vi "FPGA-7841R-Control V3.vi"(0 "Waveform Data":T4, 1 "Current Frame":u8, 2 "Action":T5=enum."Exit", 3 "Laser On Time (Ticks)":u8=13, 5 "Laser Controls":T1 {"STED Power (V)" scale=0.0..10.0}, 7 "Manual Controls":T3={"Galvo 1 Position (I16)"=-280, "Galvo 2 Position (I16)"=-280, "X Axis Voltage (I16)"=0, "Y Axis Voltage (I16)"=0, "Z Axis Voltage (I16)"=0, "Res Mirror Amp (I16)"=0, "Res Mirror Mute"=FALSE, "Upper Shutter"=FALSE, "Lower Shutter"=FALSE}, 9 "Image Acquisition Parameters":T2={"Scan Type"=enum."Sample Scanning", "Scan Mode"=enum."XY", "Fast Axis Frequency (Hz)"=100.0, "Image Format"=128, "Line Accumulations"=1, "Frames Per Capture"=1, "Frames Accumulations"=1, "Image Dimension (um)"=[], "Number of Z Steps"=1, "Z Steps Size (um)"=1.0, "Pixel Size (nm)"=[], "Customized Image Format"=[]} {"Z Steps Size (um)" min=0.0; "Number of Z Steps" min=1; "Frames Accumulations" min=1; "Frames Per Capture" min=1; "Line Accumulations" min=1; "Image Format" items=["64 x 64"=64, "128 x 128"=128, "256 x 256"=256, "512 x 512"=512, "1024 x 1024"=1024, "2048 x 2048"=2048, "Customized..."=0]}, 11 "Initialize":bool, 12 "Unused Axis Offset (I16)":i16, 14 "Laser Delay (Ticks)":u8=6) -> (4 "Shutter Status":cluster{"US Status":bool, "LS Status":bool}, 15 "Initalized":bool)   [LabVIEW 2014]
uses:
  FPGA-7842R-Reference.ctl
  Waveform Data.ctl
  Manual Controls V2.ctl
  Type Defs/Image Acquisition Parameters v2.ctl
  Laser Controls.ctl
  <vilib>/FPGAPlugInAG/PCIe-7841R/niLvFpga_Open_PCIe-7841R.vi
  <vilib>/Utility/error.llb/Error Cluster From Error Code.vi
  <vilib>/rvi/errors/niLvFpgaAdjustHostInterfaceError.vi
  <vilib>/FPGAPlugInAG/PCIe-7841R/niLvFpga_Run_PCIe-7841R.vi
  <vilib>/FPGAPlugInAG/PCIe-7841R/niLvFpga_Close_PCIe-7841R.vi
  <vilib>/rvi/interface/nirviOpenFPGA/nirviOpenFPGA.xnode
  FPGA Bitfiles/MainSTEDFPGAProj_FPGATarget_WaveformandLaser_VYICzb2jDIA.lvbitx
  FPGA Target VIs/FPGA-7841R/Waveform and Laser Controls V6.vi
  <vilib>/rvi/interface/nirviReadWriteControl/nirviReadWriteControl.xnode
  FPGA Target VIs/FPGA-7841R/Waveform Scan Parameters.ctl
  <vilib>/rvi/interface/nirviMethod/nirviMethod.xnode
  <vilib>/rvi/interface/nirviCloseFPGA/nirviCloseFPGA.xnode
  NiFpgaLv.dll
panel:
  # "Fast Axis"
  # "Slow Axis"
  # "XY"
  # "Z"
  # "Length"
  # "Height"
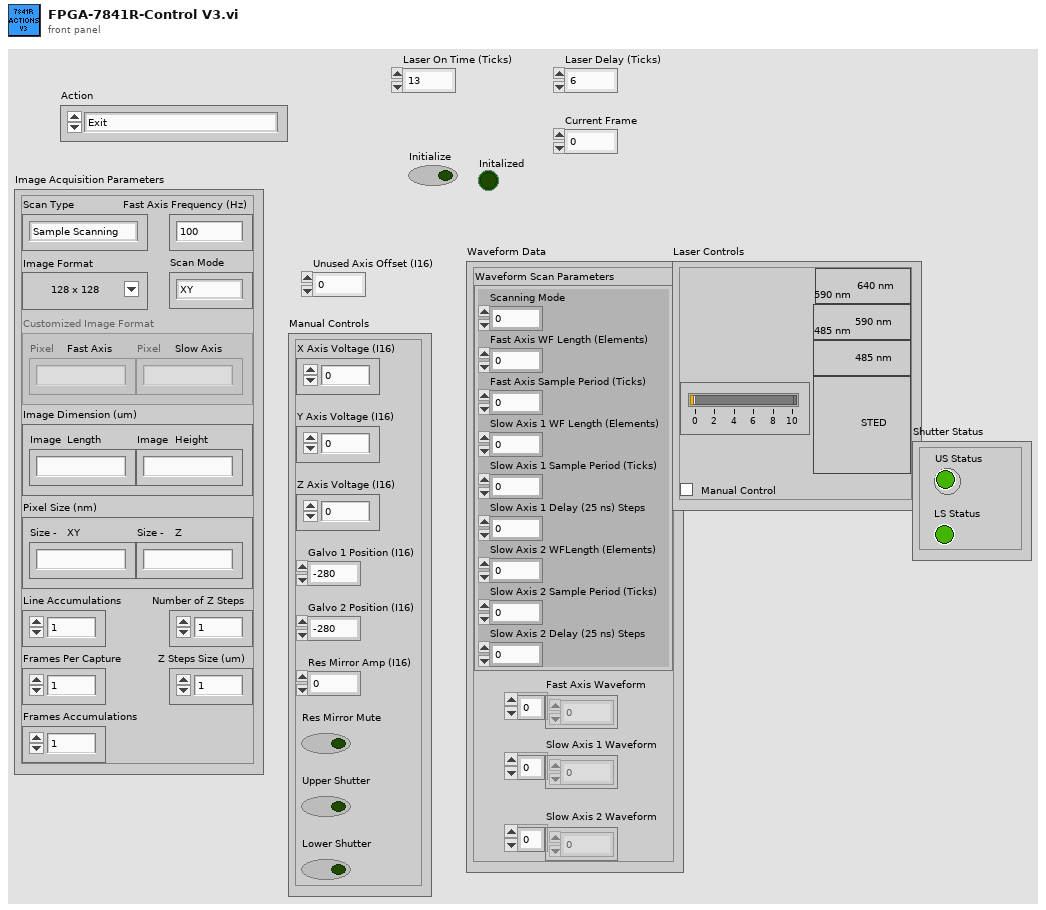
[diagram p1: front panel]
types:
  T1 = typedef "Laser Controls.ctl" = cluster{"STED Power (V)":dbl, "STED":bool, "650 nm":bool, "590 nm":bool, "485 nm":bool, "Manual Control":bool}
  T2 = typedef "Image Acquisition Parameters v2.ctl" = cluster{"Scan Type":enum16{"Sample Scanning", "Beam Scanning"}, "Scan Mode":enum16{"XY", "XZ", "YZ", "XYZ"}, "Fast Axis Frequency (Hz)":dbl, "Image Format":u16, "Line Accumulations":u16, "Frames Per Capture":u16, "Frames Accumulations":u16, "Image Dimension (um)":dbl[], "Number of Z Steps":u8, "Z Steps Size (um)":dbl, "Pixel Size (nm)":dbl[], "Customized Image Format":dbl[]}
  T3 = typedef "Manual Controls V2.ctl" = cluster{"Galvo 1 Position (I16)":i16, "Galvo 2 Position (I16)":i16, "X Axis Voltage (I16)":i16, "Y Axis Voltage (I16)":i16, "Z Axis Voltage (I16)":i16, "Res Mirror Amp (I16)":i16, "Res Mirror Mute":bool, "Upper Shutter":bool, "Lower Shutter":bool}
  T4 = typedef "Waveform Data.ctl" = cluster{"Waveform Scan Parameters":cluster{"Scanning Mode":u8, "Fast Axis WF Length (Elements)":i32, "Fast Axis Sample Period (Ticks)":u32, "Slow Axis 1 WF Length (Elements)":i32, "Slow Axis 1 Sample Period (Ticks)":u32, "Slow Axis 1 Delay (25 ns) Steps":i32, "Slow Axis 2 WFLength (Elements)":i32, "Slow Axis 2 Sample Period (Ticks)":u32, "Slow Axis 2 Delay (25 ns) Steps":i32}, "Fast Axis Waveform":dbl[], "Slow Axis 1 Waveform":dbl[], "Slow Axis 2 Waveform":dbl[]}
  T5 = typedef "FPGA-7842R-Reference.ctl" = enum16{"Stage Control", "Laser Control", "Unused Axis I16", "Exit", "Set Res Mirror", "Set Galvo", "Current Frame for Capture", "Default", "Close FPGA", "Stop Waveforms", "Start Waveforms", "Shutter Control", "Initialize"}
  T6 = cluster{"Scanning Mode":u8, "Fast Axis WF Length (Elements)":i32, "Fast Axis Sample Period (Ticks)":u32, "Slow Axis 1 WF Length (Elements)":i32, "Slow Axis 1 Sample Period (Ticks)":u32, "Slow Axis 1 Delay (25 ns) Steps":i32, "Slow Axis 2 WFLength (Elements)":i32, "Slow Axis 2 Sample Period (Ticks)":u32, "Slow Axis 2 Delay (25 ns) Steps":i32}
  T7 = cluster{"Res Mirror Amp (I16)":i16, "Res Mirror Mute":bool}
  T8 = typedef "Scan Parameters.ctl" = cluster{"Fast_Ax_Amp_V":dbl, "Fast_Ax_Off_V":dbl, "Slow_Ax_Amp_V":dbl, "Slow_Ax_Off_V ":dbl, "Slow_Ax_Max_V_VperS":dbl, "Slow_Ax1_Del25ns":i32, "Slow_Ax2_Del25ns":i32, "Stage_X_Off_V":dbl, "Stage_Y_Off_V":dbl, "Stage_Z_Off_V":dbl, "Galvo1_Off_V":dbl, "Galvo2_Off_V":dbl, "Last_Scan_Mode":enum16{"XY", "XZ", "YZ", "XYZ"}, "Current_Scan_Mode":enum16{"XY", "XZ", "YZ", "XYZ"}, "Fly_Back_Lines":u16, "Linear_Ramp_End":u32, "Z_Step_I16":i16, "Z_Start_I16":i16, "Laser_States _U32":u32, "590_Voltage_I16":i16, "775_AOM_Volt_I16":i16, "Blanking OFF":bool, "Unused_Axis_I16":i16}
  T9 = cluster{"Upper Shutter Status":bool, "Lower Shutter Status":bool}
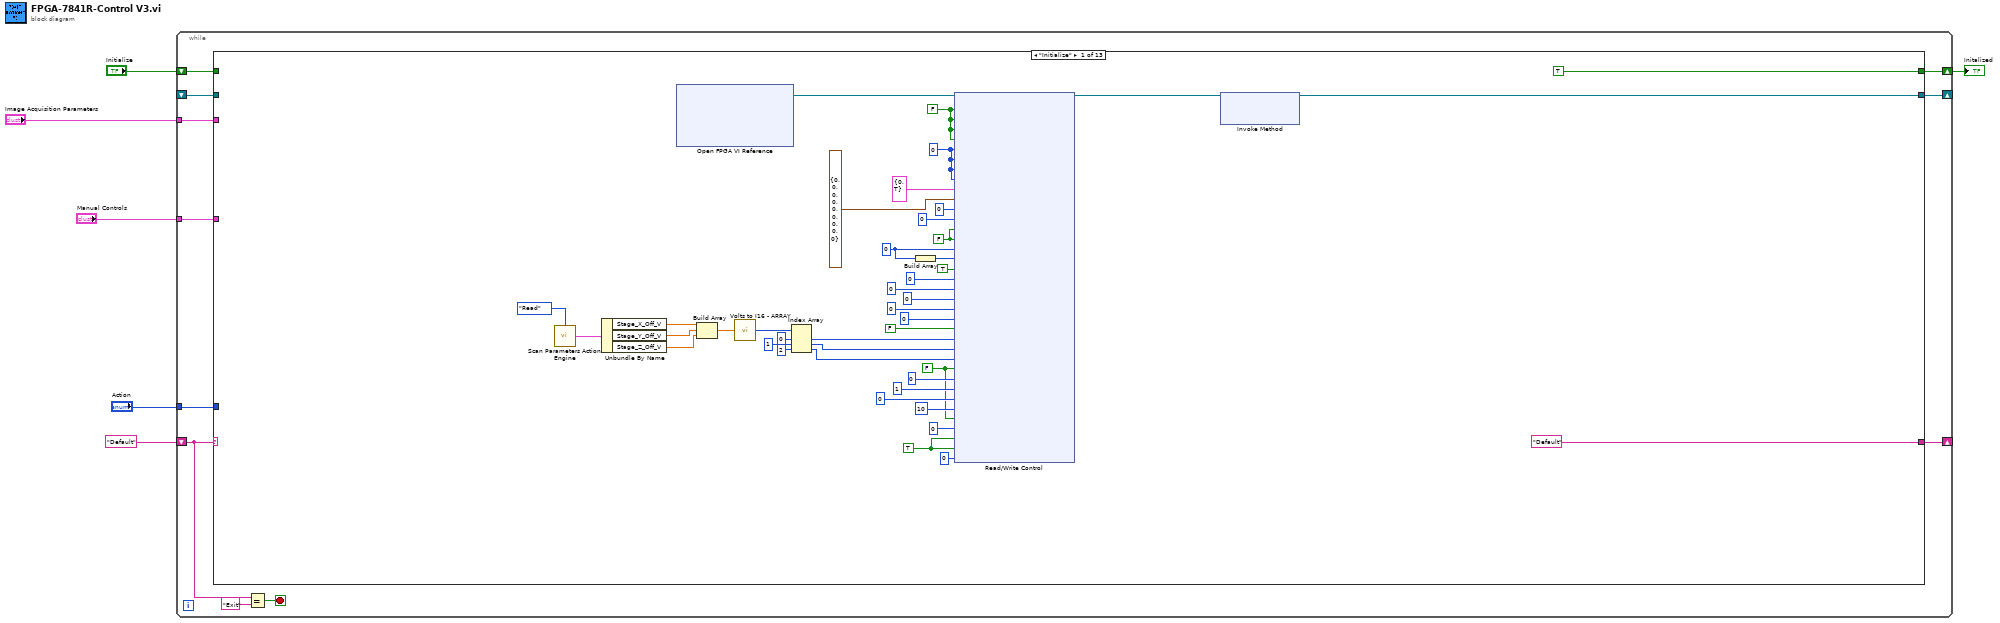
[diagram p0: block diagram]
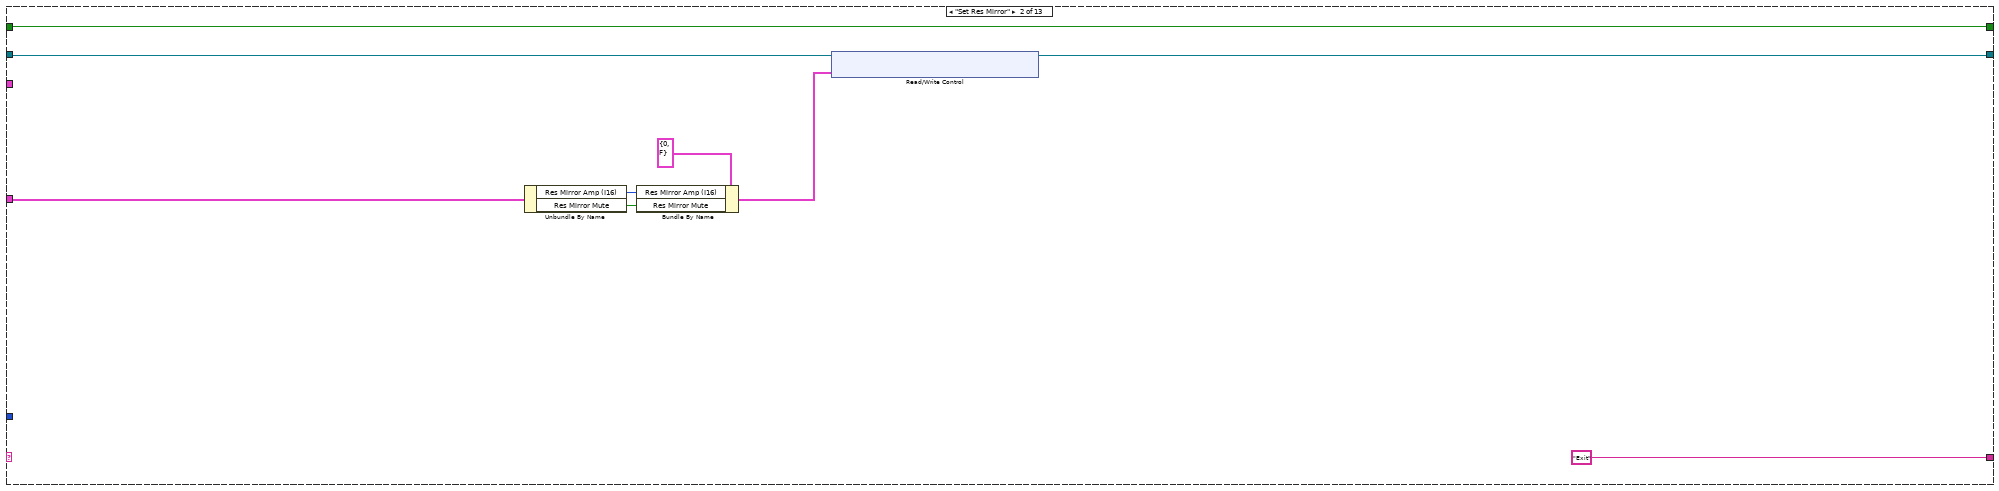
[diagram p2: hidden frame]
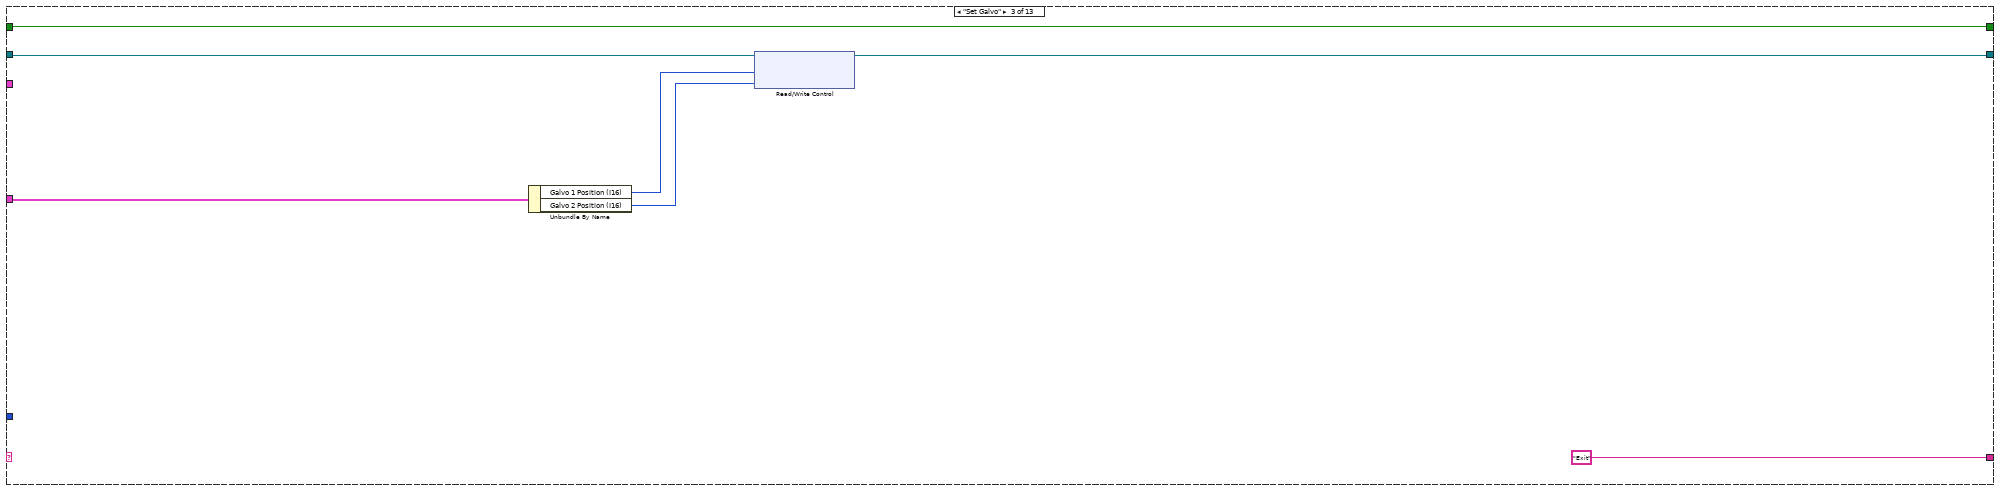
[diagram p3: hidden frame]
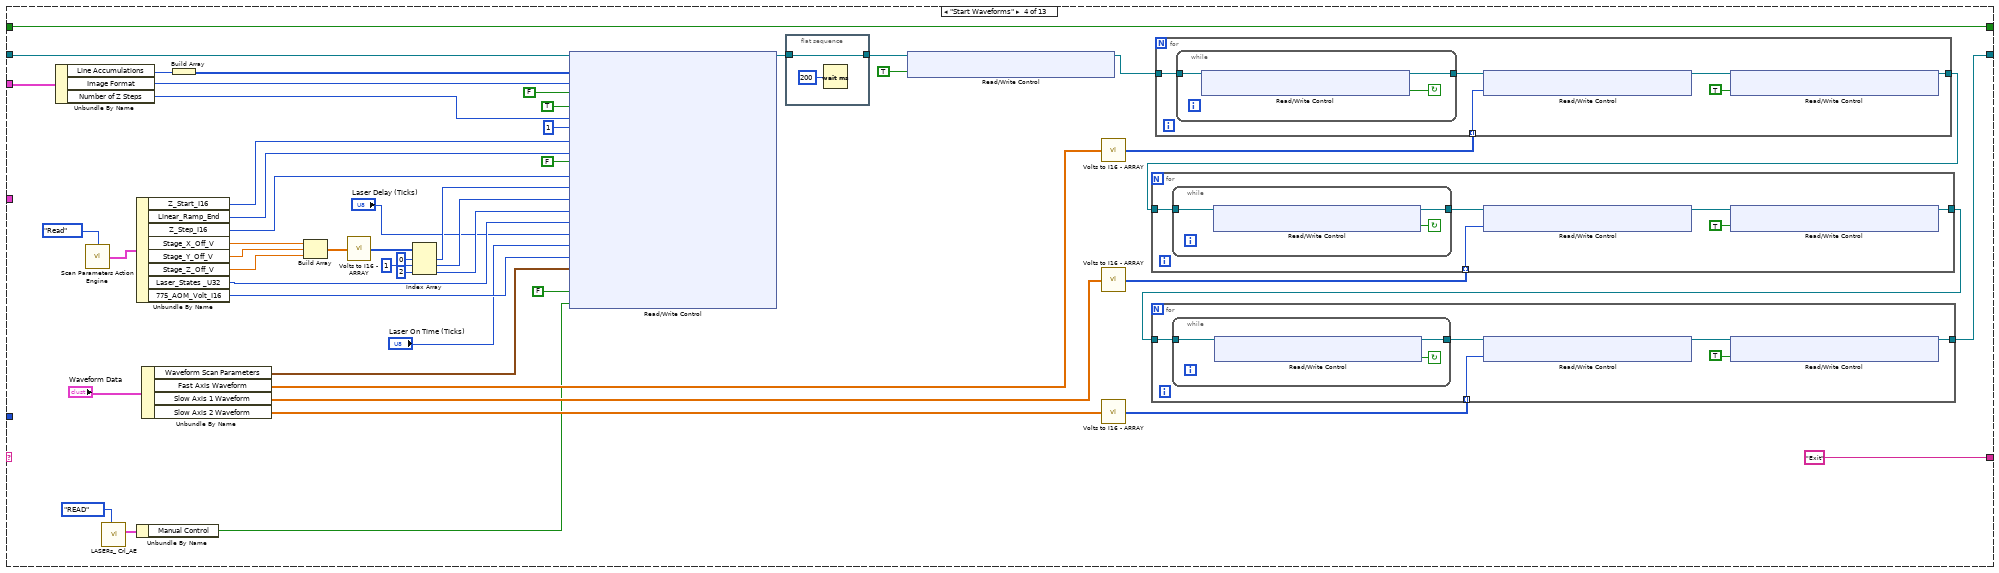
[diagram p4: hidden frame]
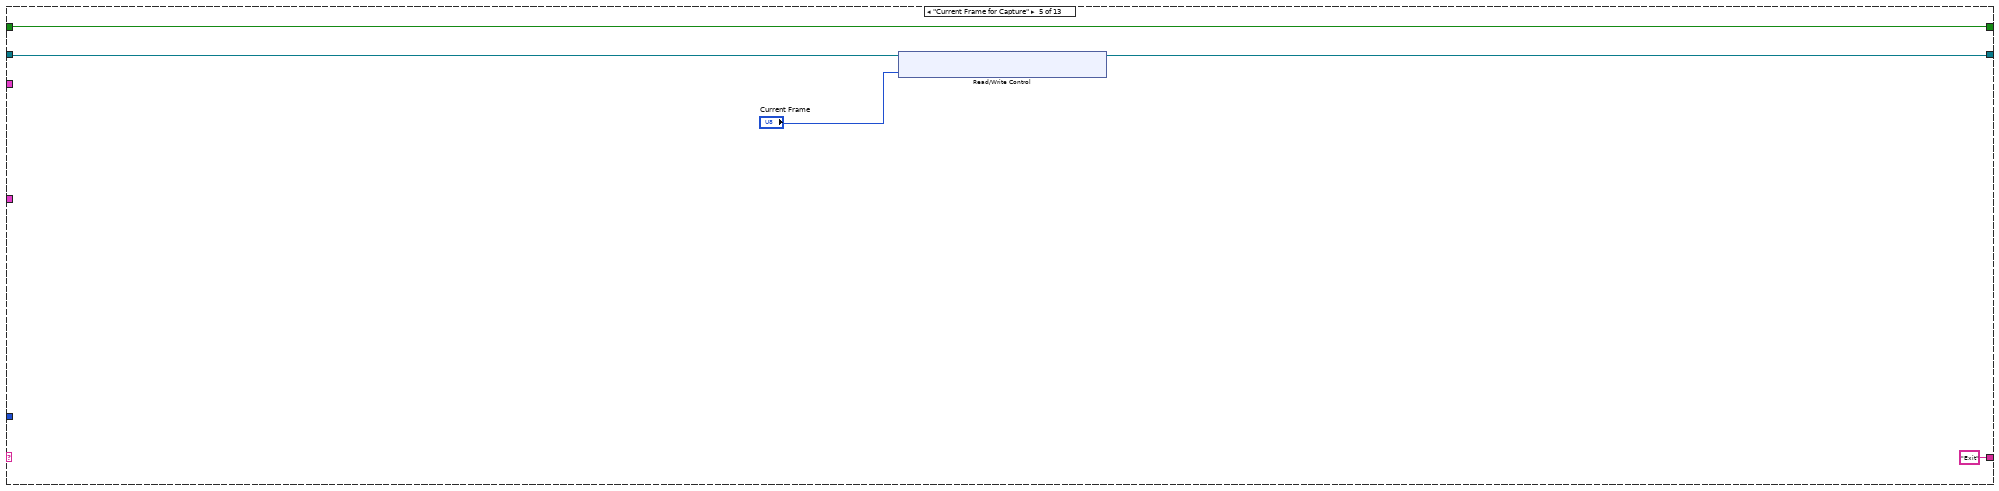
[diagram p5: hidden frame]
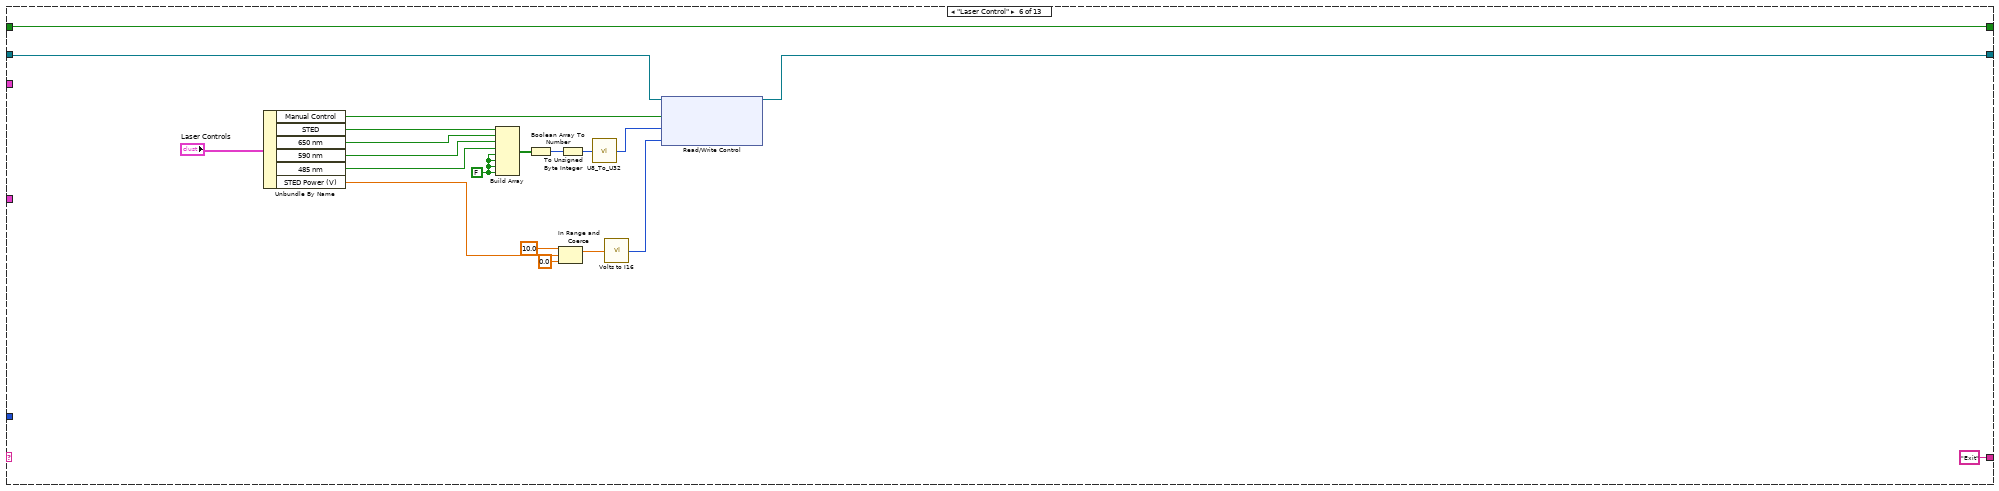
[diagram p6: hidden frame]
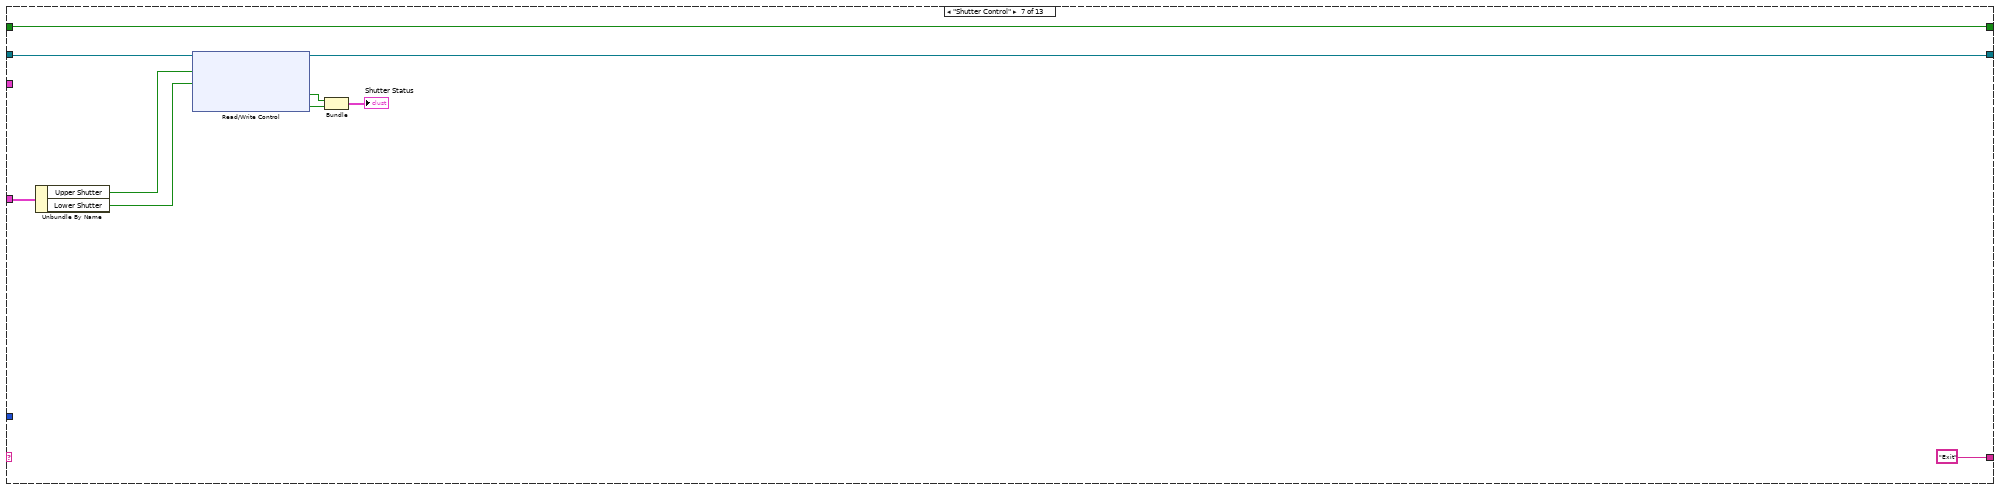
[diagram p7: hidden frame]
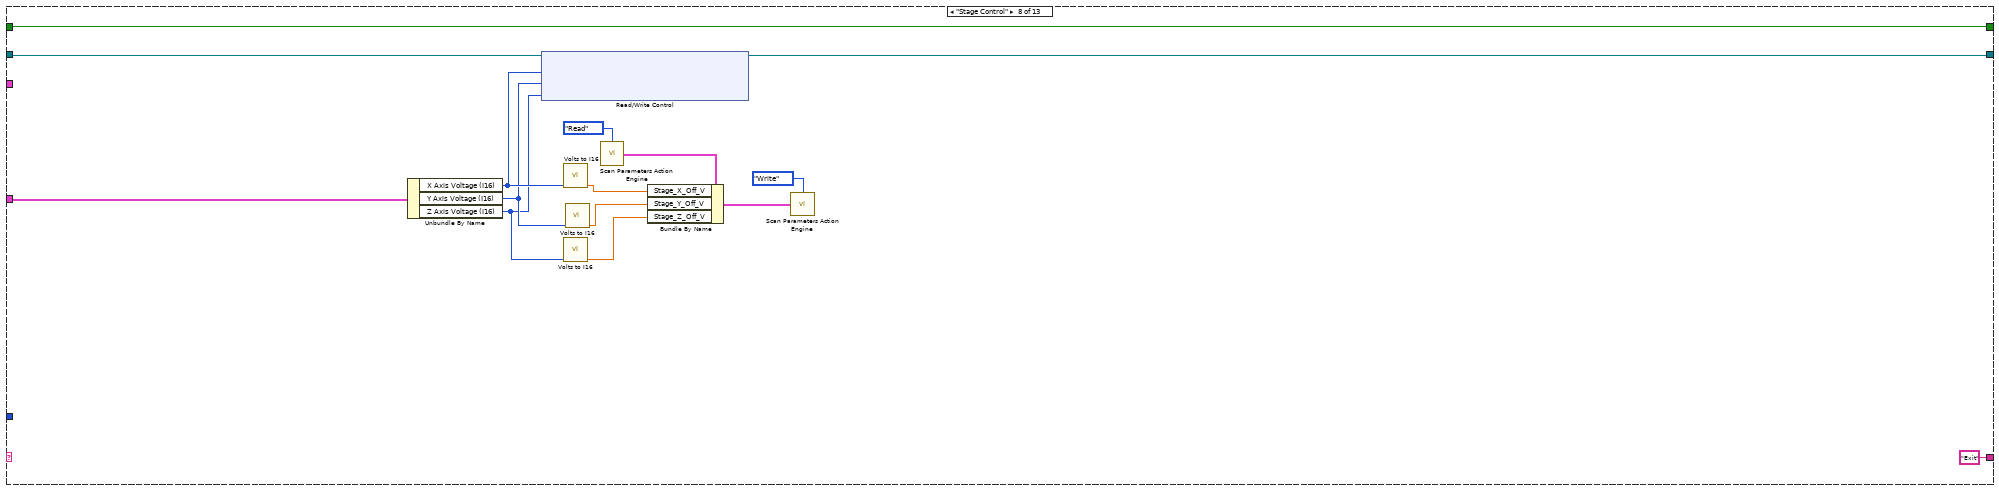
[diagram p8: hidden frame]
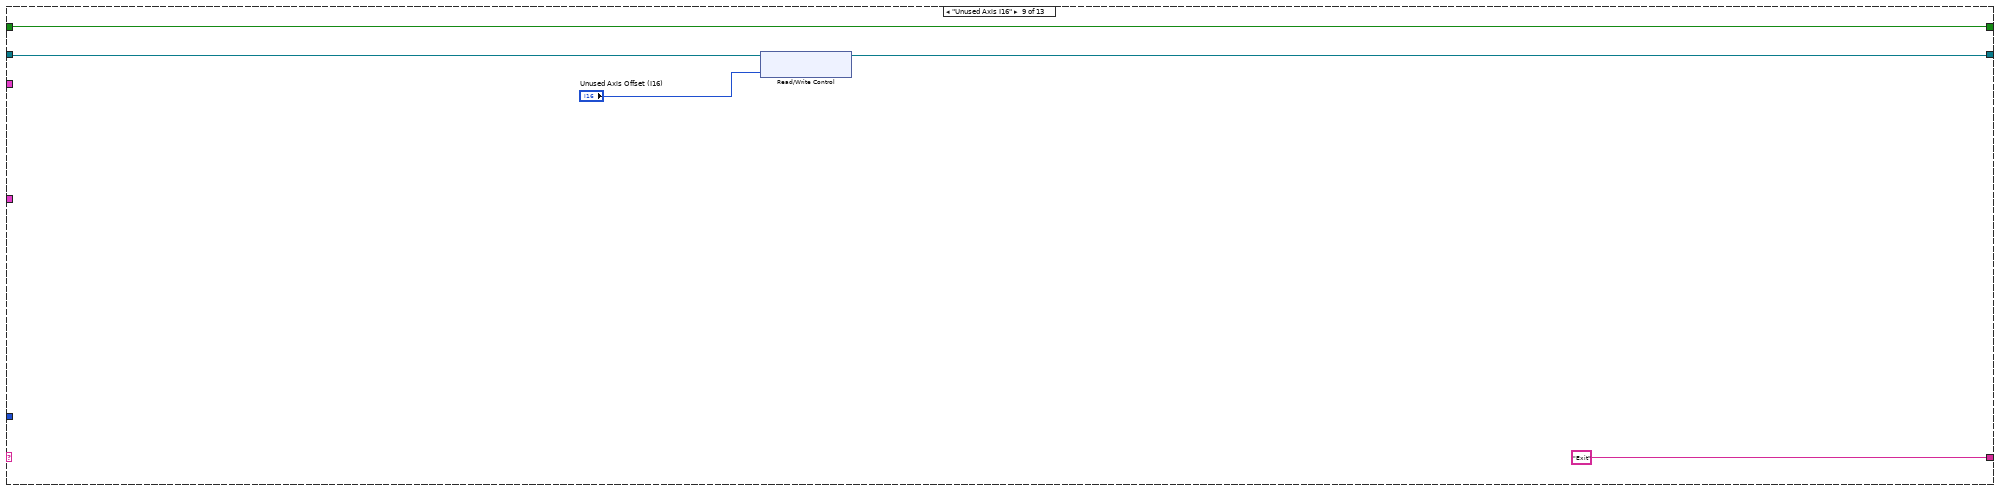
[diagram p9: hidden frame]
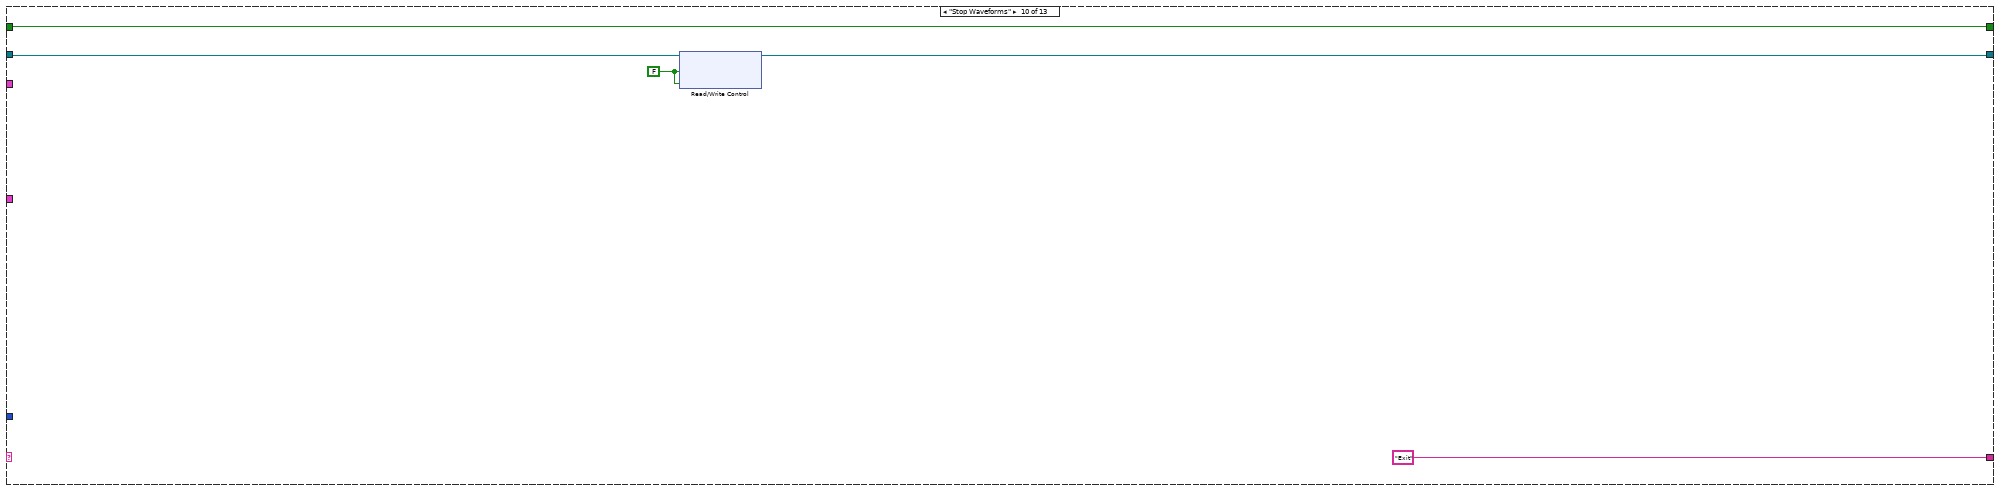
[diagram p10: hidden frame]
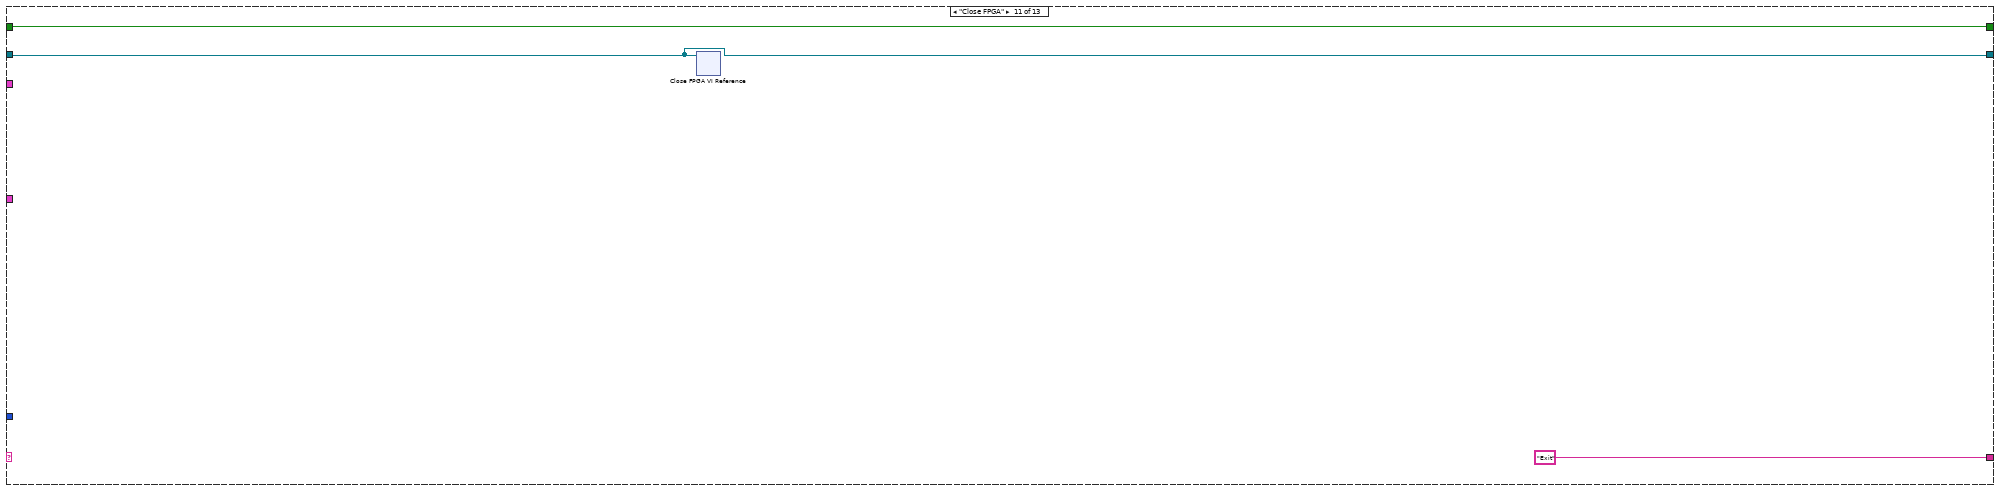
[diagram p11: hidden frame]
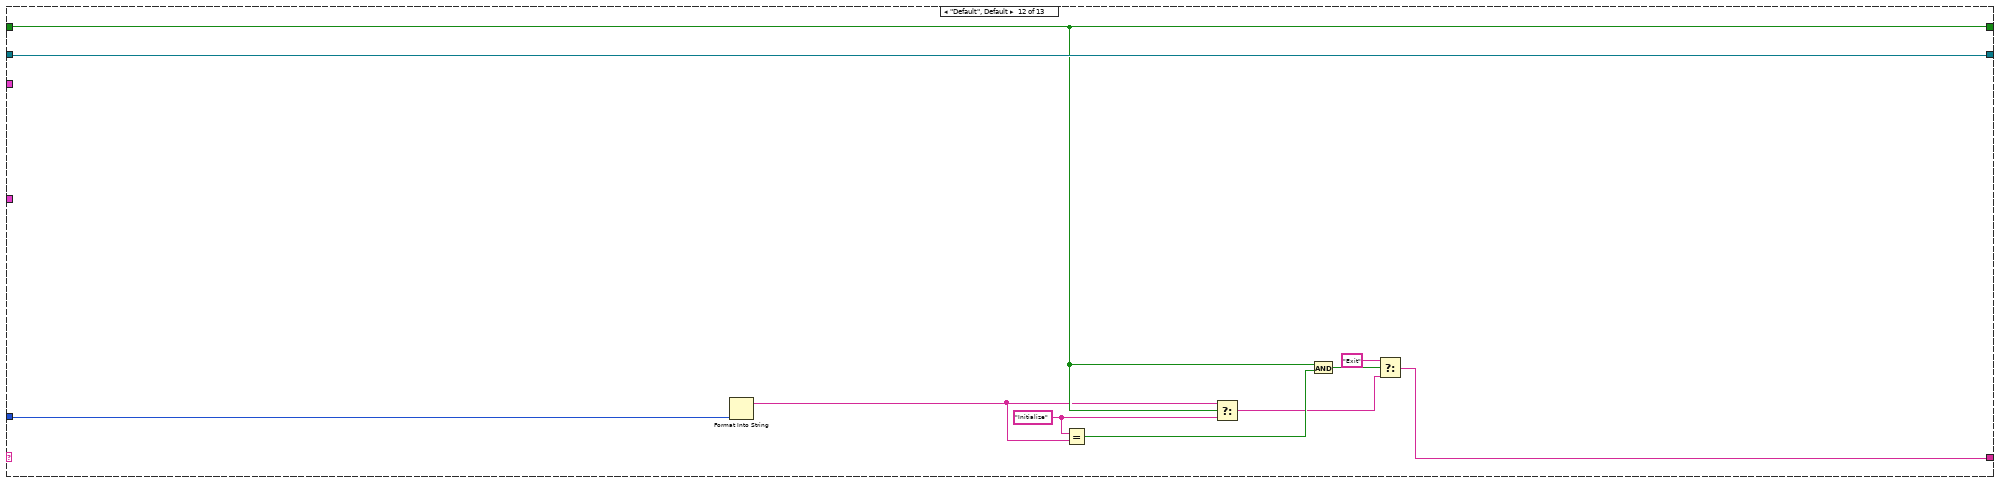
[diagram p12: hidden frame]
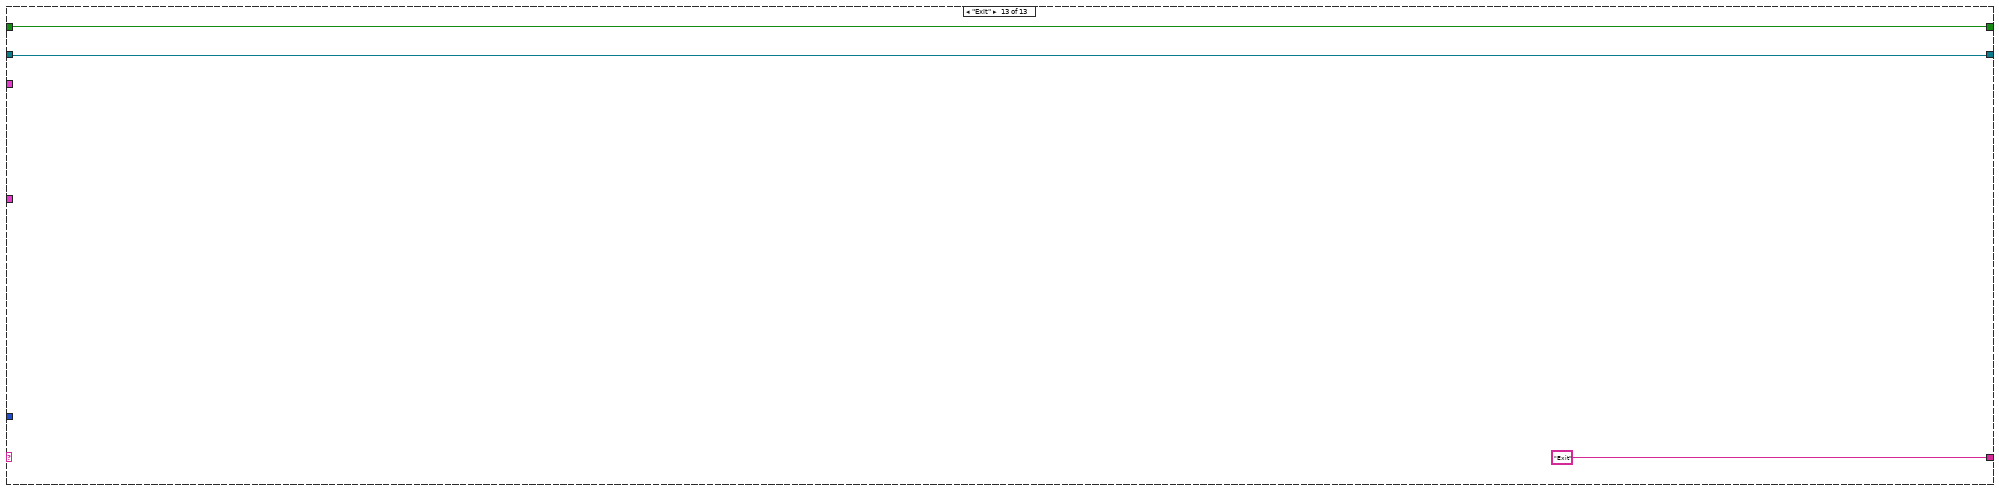
[diagram p13: hidden frame]
diagram:
  n1 = while {
    shift-right: [w17] -> _
    shift-left: _ -> [w16]
    shift-right: [w14] -> _
    shift-left: "Default" -> [w13]
    tunnel: "Action" -> [w15]
    shift-right: [w10] -> w3
    shift-left: "Initialize" -> [w9]
    tunnel: "Manual Controls" -> [w8]
    tunnel: "Image Acquisition Parameters" -> [w7]
    stop <- w11 stop-if-true
    n2 = case shown="\"Initialize\"" w13 {
      tunnel: [w50 w65 w72 w115 w158 w176 w188 w201 w207 w214 w216 w228 w230] -> w17
      tunnel: w16 -> [_ w66 w73 w118 w159 w177 w189 w202 w208 w215 w216 w228 w230]
      tunnel: w15 -> [_ _ _ _ _ _ _ _ _ _ _ w227 _]
      tunnel: ["Default" ("f") "Exit" ("f") "Exit" ("f") "Exit" ("f") "Exit" ("f") "Exit" ("f") "Exit" ("f") "Exit" ("f") "Exit" ("f") "Exit" ("f") "Exit" ("f") w221 "Exit" ("f")] -> w14
      tunnel: [TRUE w68 w75 w120 w160 w179 w190 w204 w210 w213 w218 w226 w231] -> w10
      tunnel: w9 -> [_ w68 w75 w120 w160 w179 w190 w204 w210 w213 w218 w226 w231]
      tunnel: w8 -> [_ w64 w71 _ _ _ w183 w203 _ _ _ _ _]
      tunnel: w7 -> [_ _ _ w109 _ _ _ _ _ _ _ _ _]
      frame "Initialize" {
        w19 = TRUE ("Upper Shutter Command")
        w21 = FALSE ("Blanking Off/Manual")
        w46 = u16 0 ("Number of Lines")
        w48 = FALSE ("Reset Position Error")
        w59 = i16 0 ("Fast Axis Waveform Element")
        w58 = FALSE ("WF 1 Data Loaded")
        n3 = call "Scan Parameters Action Engine.vi"("Action"=enum16{"Read", "Write"}."Read") -> ("Scan Parameters OUT"=w37:T8)  [unwired: 14 in]
        n4 = Unbundle By Name(w37) -> ("Stage_X_Off_V"=w36:dbl, "Stage_Y_Off_V"=w34:dbl, "Stage_Z_Off_V"=w35:dbl)
        n5 = xnode "Open FPGA VI Reference"() -> ("FPGA VI Reference Out"=w49:refnum<k20>)  [unwired: 2 in, 1 out]
        n6 = Build Array(w36, w34, w35) -> (w33:dbl[])
        n7 = call "Volts to I16 - ARRAY.vi"("Voltage (V)"=w33) -> ("I16"=w32:i16[])  [unwired: 14 in]
        n8 = Index Array(array=w32, index #1=0 ("index"), index #2=1 ("index"), index #3=2 ("index")) -> (element #1=w28:i16, element #2=w26:i16, element #3=w27:i16)
        n9 = Build Array(w46) -> (w45:u16[])
        n10 = xnode "Read/Write Control"("FPGA VI Reference In"=w49, "WF 1 Data Loaded"=w58, "WF 2 Data Loaded"=w58, "WF 3 Data Loaded"=w58, "Start Waveforms"=w58, "Fast Axis Waveform Element"=w59, "Slow Axis 1 Waveform Element"=w59, "Slow Axis 2 Waveform Element"=w59, "Unused Axis Offset"=w59, "Resonant Mirror"=T7 {"Res Mirror Amp (I16)"=0, "Res Mirror Mute"=TRUE} ("Resoance Mirror"), "Waveform Scan Parameters"=T6 {"Scanning Mode"=0, "Fast Axis WF Length (Elements)"=0, "Fast Axis Sample Period (Ticks)"=0, "Slow Axis 1 WF Length (Elements)"=0, "Slow Axis 1 Sample Period (Ticks)"=0, "Slow Axis 1 Delay (25 ns) Steps"=0, "Slow Axis 2 WFLength (Elements)"=0, "Slow Axis 2 Sample Period (Ticks)"=0, "Slow Axis 2 Delay (25 ns) Steps"=0}, "Galvo 2 Position (I16)"=i16 0, "Galvo 1 Position (I16)"=i16 0, "Reset Position Error"=w48, "Frame Trigger"=w48, "Number of Lines"=w46, "Accums Per Line"=w45, "Stop Sync Signal"=TRUE, "Z Step Size (I16)"=i16 0, "Number of Z Steps"=u8 0, "Frames Per Z Step"=u8 0, "Z Stack Start Position (I16)"=i16 0, "End of Linear Ramp"=u32 0, "End Linear Ramp"=FALSE, "X Piezo Axis"=w28, "Y Piezo Axis"=w26, "Z Piezo Axis"=w27, "Blanking Off/Manual"=w21, "Laser States"=u32 0, "Laser Delay (Ticks)"=u8 1, "Sequences"=u8 0, "Laser On Time (Ticks)"=u8 10, "Laser Blank Trigger"=w21, "775 AOM (I16)"=i16 0 ("590 Analog Voltage (I16)"), "Upper Shutter Command"=w19, "Lower Shutter Command"=w19, "Current Frame"=u8 0) -> ("FPGA VI Reference Out"=w55:refnum<k20>)  [unwired: 1 in, 1 out]
        n11 = xnode "Invoke Method"("FPGA VI Reference In"=w55) -> ("FPGA VI Reference Out"=w50:refnum<k20>)  [unwired: 2 in, 1 out]
      }
      frame "Set Res Mirror" {
        n12 = Unbundle By Name(w64) -> ("Res Mirror Amp (I16)"=w63:i16, "Res Mirror Mute"=w62:bool)
        n13 = Bundle By Name(cluster=T7 {"Res Mirror Amp (I16)"=0, "Res Mirror Mute"=FALSE} ("Resoance Mirror"), "Res Mirror Amp (I16)"=w63, "Res Mirror Mute"=w62) -> (w60:T7)
        n14 = xnode "Read/Write Control"("FPGA VI Reference In"=w66, "Resonant Mirror"=w60) -> ("FPGA VI Reference Out"=w65:refnum<k20>)  [unwired: 1 in, 1 out]
      }
      frame "Set Galvo" {
        n15 = Unbundle By Name(w71) -> ("Galvo 1 Position (I16)"=w70:i16, "Galvo 2 Position (I16)"=w69:i16)
        n16 = xnode "Read/Write Control"("FPGA VI Reference In"=w73, "Galvo 1 Position (I16)"=w70, "Galvo 2 Position (I16)"=w69) -> ("FPGA VI Reference Out"=w72:refnum<k20>)  [unwired: 1 in, 1 out]
      }
      frame "Start Waveforms" {
        n17 = Unbundle By Name(w109) -> ("Line Accumulations"=w107:u16, "Image Format"=w108:u16, "Number of Z Steps"=w98:u8)
        n18 = call "Scan Parameters Action Engine.vi"("Action"=enum16{"Read", "Write"}."Read") -> ("Scan Parameters OUT"=w102:T8)  [unwired: 14 in]
        n19 = call "LASERs_ Crl_AE.vi"("Action"=enum16{"READ", "WRITE"}."READ") -> ("Detectors Parameters Out"=w77:T1)  [unwired: 10 in]
        n20 = Unbundle By Name(w102) -> ("Z_Start_I16"=w100:i16, "Linear_Ramp_End"=w101:u32, "Z_Step_I16"=w97:i16, "Stage_X_Off_V"=w90:dbl, "Stage_Y_Off_V"=w89:dbl, "Stage_Z_Off_V"=w88:dbl, "Laser_States _U32"=w84:u32, "775_AOM_Volt_I16"=w83:i16)
        n21 = Unbundle By Name(w77) -> ("Manual Control"=w76:bool)
        n22 = Unbundle By Name("Waveform Data") -> ("Waveform Scan Parameters"=w82:T6, "Fast Axis Waveform"=w122:dbl[], "Slow Axis 1 Waveform"=w114:dbl[], "Slow Axis 2 Waveform"=w121:dbl[])
        n23 = Build Array(w107) -> (w106:u16[])
        n24 = Build Array(w90, w89, w88) -> (w95:dbl[])
        n25 = call "Volts to I16 - ARRAY.vi"("Voltage (V)"=w95) -> ("I16"=w94:i16[])  [unwired: 14 in]
        n26 = Index Array(array=w94, index #1=0 ("index"), index #2=1 ("index"), index #3=2 ("index")) -> (element #1=w87:i16, element #2=w86:i16, element #3=w85:i16)
        n27 = xnode "Read/Write Control"("FPGA VI Reference In"=w118, "Accums Per Line"=w106, "Number of Lines"=w108, "Frame Trigger"=FALSE, "Stop Sync Signal"=TRUE, "Number of Z Steps"=w98, "Frames Per Z Step"=u8 1, "Z Stack Start Position (I16)"=w100, "End of Linear Ramp"=w101, "End Linear Ramp"=FALSE, "Z Step Size (I16)"=w97, "X Piezo Axis"=w87, "Y Piezo Axis"=w86, "Z Piezo Axis"=w85, "Laser States"=w84, "Laser Delay (Ticks)"="Laser Delay (Ticks)", "Laser On Time (Ticks)"="Laser On Time (Ticks)", "775 AOM (I16)"=w83, "Waveform Scan Parameters"=w82, "Frame Trigger"=FALSE, "Blanking Off/Manual"=w76) -> ("FPGA VI Reference Out"=w116:refnum<k20>)  [unwired: 1 in, 2 out]
        n28 = flat-sequence {
          tunnel: [w128] -> w117
          tunnel: w116 -> [w128]
          frame #0 {
            n29 = Wait (ms)(milliseconds to wait=u32 200) -> ()  [unwired: 1 out]
          }
        }
        n30 = xnode "Read/Write Control"("FPGA VI Reference In"=w117, "Start Waveforms"=TRUE) -> ("FPGA VI Reference Out"=w123:refnum<k20>)  [unwired: 1 in, 1 out]
        n31 = call "Volts to I16 - ARRAY.vi"("Voltage (V)"=w122) -> ("I16"=w126:i16[])  [unwired: 14 in]
        n32 = call "Volts to I16 - ARRAY.vi"("Voltage (V)"=w114) -> ("I16"=w112:i16[])  [unwired: 14 in]
        n33 = call "Volts to I16 - ARRAY.vi"("Voltage (V)"=w121) -> ("I16"=w113:i16[])  [unwired: 14 in]
        n34 = for {
          tunnel: w123 -> [w151]
          tunnel: [w149] -> w125
          tunnel: w126 -> [w147] mode=indexing
          n35 = while {
            tunnel: w151 -> [w155]
            tunnel: [w154] -> w150
            stop <- w153 continue-if-true
            n36 = xnode "Read/Write Control"("FPGA VI Reference In"=w155) -> ("FPGA VI Reference Out"=w154:refnum<k20>, "WF 1 Data Loaded"=w153:bool)  [unwired: 1 in, 1 out]
          }
          n37 = xnode "Read/Write Control"("FPGA VI Reference In"=w150, "Fast Axis Waveform Element"=w147) -> ("FPGA VI Reference Out"=w152:refnum<k20>)  [unwired: 1 in, 1 out]
          n38 = xnode "Read/Write Control"("FPGA VI Reference In"=w152, "WF 1 Data Loaded"=TRUE ("Host Data Loaded")) -> ("FPGA VI Reference Out"=w149:refnum<k20>)  [unwired: 1 in, 1 out]
        }
        n39 = for {
          tunnel: w125 -> [w142]
          tunnel: [w140] -> w96
          tunnel: w112 -> [w138] mode=indexing
          n40 = while {
            tunnel: w142 -> [w146]
            tunnel: [w145] -> w141
            stop <- w144 continue-if-true
            n41 = xnode "Read/Write Control"("FPGA VI Reference In"=w146) -> ("FPGA VI Reference Out"=w145:refnum<k20>, "WF 2 Data Loaded"=w144:bool)  [unwired: 1 in, 1 out]
          }
          n42 = xnode "Read/Write Control"("FPGA VI Reference In"=w141, "Slow Axis 1 Waveform Element"=w138) -> ("FPGA VI Reference Out"=w143:refnum<k20>)  [unwired: 1 in, 1 out]
          n43 = xnode "Read/Write Control"("FPGA VI Reference In"=w143, "WF 2 Data Loaded"=TRUE ("Host Data Loaded")) -> ("FPGA VI Reference Out"=w140:refnum<k20>)  [unwired: 1 in, 1 out]
        }
        n44 = for {
          tunnel: w96 -> [w133]
          tunnel: [w131] -> w115
          tunnel: w113 -> [w129] mode=indexing
          n45 = while {
            tunnel: w133 -> [w137]
            tunnel: [w136] -> w132
            stop <- w135 continue-if-true
            n46 = xnode "Read/Write Control"("FPGA VI Reference In"=w137) -> ("FPGA VI Reference Out"=w136:refnum<k20>, "WF 3 Data Loaded"=w135:bool)  [unwired: 1 in, 1 out]
          }
          n47 = xnode "Read/Write Control"("FPGA VI Reference In"=w132, "Slow Axis 2 Waveform Element"=w129) -> ("FPGA VI Reference Out"=w134:refnum<k20>)  [unwired: 1 in, 1 out]
          n48 = xnode "Read/Write Control"("FPGA VI Reference In"=w134, "WF 3 Data Loaded"=TRUE ("Host Data Loaded")) -> ("FPGA VI Reference Out"=w131:refnum<k20>)  [unwired: 1 in, 1 out]
        }
      }
      frame "Current Frame for Capture" {
        n49 = xnode "Read/Write Control"("FPGA VI Reference In"=w159, "Current Frame"="Current Frame") -> ("FPGA VI Reference Out"=w158:refnum<k20>)  [unwired: 1 in, 1 out]
      }
      frame "Laser Control" {
        w170 = FALSE ("element")
        n50 = Unbundle By Name("Laser Controls") -> ("Manual Control"=w178:bool, "STED"=w167:bool, "650 nm"=w166:bool, "590 nm"=w165:bool, "485 nm"=w164:bool, "STED Power (V)"=w163:dbl)
        n51 = Build Array(w167, w166, w165, w164, w170, w170, w170, w170) -> (w168:bool[])
        n52 = Boolean Array To Number(Boolean array=w168) -> (number=w169:u32)
        n53 = In Range and Coerce(upper limit=10.0, x=w163, lower limit=0.0) -> (coerced(x)=w174:dbl)  [unwired: 1 out]
        n54 = To Unsigned Byte Integer(number=w169) -> (unsigned 8bit integer=w171:u8)
        n55 = call "U8_To_U32.vi"("U8 IN"=w171) -> ("U32 OUT"=w162:u32)  [unwired: 13 in, 1 out]
        n56 = call "Volts to I16.vi"("Voltage (V)"=w174) -> ("I16"=w161:i16)  [unwired: 13 in, 1 out]
        n57 = xnode "Read/Write Control"("FPGA VI Reference In"=w177, "Blanking Off/Manual"=w178, "Laser States"=w162, "775 AOM (I16)"=w161) -> ("FPGA VI Reference Out"=w176:refnum<k20>)  [unwired: 1 in, 1 out]
      }
      frame "Shutter Control" {
        n58 = Unbundle By Name(w183) -> ("Upper Shutter"=w181:bool, "Lower Shutter"=w182:bool)
        n59 = xnode "Read/Write Control"("FPGA VI Reference In"=w189, "Upper Shutter Command"=w181, "Lower Shutter Command"=w182) -> ("FPGA VI Reference Out"=w188:refnum<k20>, "Upper Shutter Status"=w186:bool, "Lower Shutter Status"=w185:bool)  [unwired: 1 in, 1 out]
        n60 = Bundle("Upper Shutter Status"=w186, "Lower Shutter Status"=w185) -> (→"Shutter Status":T9)  [unwired: 1 in]
      }
      frame "Stage Control" {
        n61 = Unbundle By Name(w203) -> ("X Axis Voltage (I16)"=w198:i16, "Y Axis Voltage (I16)"=w194:i16, "Z Axis Voltage (I16)"=w193:i16)
        n62 = xnode "Read/Write Control"("FPGA VI Reference In"=w202, "X Piezo Axis"=w198, "Y Piezo Axis"=w194, "Z Piezo Axis"=w193) -> ("FPGA VI Reference Out"=w201:refnum<k20>)  [unwired: 1 in, 1 out]
        n63 = call "Volts to I16.vi"("Volatge (I16)"=w198) -> ("Voltage (V)"=w197:dbl)  [unwired: 13 in, 1 out]
        n64 = call "Volts to I16.vi"("Volatge (I16)"=w193) -> ("Voltage (V)"=w195:dbl)  [unwired: 13 in, 1 out]
        n65 = call "Volts to I16.vi"("Volatge (I16)"=w194) -> ("Voltage (V)"=w196:dbl)  [unwired: 13 in, 1 out]
        n66 = call "Scan Parameters Action Engine.vi"("Action"=enum16{"Read", "Write"}."Read") -> ("Scan Parameters OUT"=w199:T8)  [unwired: 14 in]
        n67 = Bundle By Name(cluster=w199, "Stage_X_Off_V"=w197, "Stage_Y_Off_V"=w196, "Stage_Z_Off_V"=w195) -> (w191:T8)
        n68 = call "Scan Parameters Action Engine.vi"("Action"=enum16{"Read", "Write"}."Write", "Scan Parameters IN"=w191) -> ()  [unwired: 13 in, 1 out]
      }
      frame "Unused Axis I16" {
        n69 = xnode "Read/Write Control"("FPGA VI Reference In"=w208, "Unused Axis Offset"="Unused Axis Offset (I16)") -> ("FPGA VI Reference Out"=w207:refnum<k20>)  [unwired: 1 in, 1 out]
      }
      frame "Stop Waveforms" {
        w211 = FALSE ("Start Waveforms")
        n70 = xnode "Read/Write Control"("FPGA VI Reference In"=w215, "Start Waveforms"=w211, "Stop Sync Signal"=w211) -> ("FPGA VI Reference Out"=w214:refnum<k20>)  [unwired: 1 in, 1 out]
      }
      frame "Close FPGA" {
        n71 = xnode "Close FPGA VI Reference"("FPGA VI Reference In"=w216) -> ()  [unwired: 1 in, 1 out]
      }
      frame "Default", Default {
        w220 = "Initialize" ("f")
        n72 = Format Into String(w227) -> (resulting string=w219:string)  [unwired: 3 in, 1 out]
        n73 = Equal?(x=w220, y=w219) -> (x = y?=w225:bool)
        n74 = Select(t=w219, s=w226, f=w220) -> (s? t:f=w222:string)
        n75 = And(x=w226, y=w225) -> (x .and. y?=w224:bool)
        n76 = Select(t="Exit" ("y"), s=w224, f=w222) -> (s? t:f=w221:string)
      }
      frame "Exit" {
      }
    }
    n77 = Equal?(x=w13, y="Exit") -> (x = y?=w11:bool)
  }
  "Initalized" <- w3
